vi "LengthSqr.vi"(1 "Vec2 in":refnum<class "Vector2.lvclass">) -> (0 "Length Sqr out":sgl)   [LabVIEW 2022 SP3, in "Vector2.lvclass"]
uses:
  Vector2.lvclass
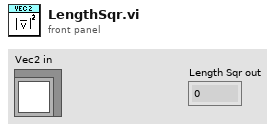
[diagram p1: front panel]
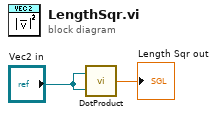
[diagram p0: block diagram]
diagram:
  n1 = call "DotProduct.vi"("Vec2 b in"="Vec2 in", "Vec2 a in"="Vec2 in") -> ("Product out"=→"Length Sqr out":sgl)
